vi "tb_01-x.vi"(0 "Etude":T2, 1 "Aff ?":bool, 5 "VS":T4, 7 "ent-2D":string[][](array[string]), 9 "do-2D":string[][](array[string]), 11 "tb in ?":bool[](array[boolean])) -> (4 "Etude":T2, 6 "VS":T4, 8 "ent-2D":T1[][](array[typedef]), 10 "do-2D":string[][](array[string]), 12 "X":string[](array[string]), 13 "X-ent":T1, 14 "X-lib":T1, 15 "tb in ?":bool[](array[boolean]))   [LabVIEW 2010, in "lv_04.lvlib"]
uses:
  lv_04/lv_04.lvlib
  lv_04/commandes/cX.ctl
  lv_04/commandes/cSTA_varid.ctl
  lv_04/commandes/c_TDMS_ch_variable.ctl
  lv_04/commandes/c_TDMS_ch_donnees.ctl
  lv_04/commandes/c0-var-n.ctl
  lv_04/commandes/cSTA_num_do_cr.ctl
  lv_04/commandes/c02-do-num.ctl
  lv_04/commandes/c04-stat-num.ctl
  lv_04/commandes/cSTA_txt_do_cr.ctl
  lv_04/commandes/c02-do-txt.ctl
  lv_04/commandes/c04-stat-txt.ctl
  lv_04/commandes/cSTA_dist.ctl
  lv_04/commandes/c03-dist-S.ctl
  lv_04/commandes/c0-dist-xy.ctl
  lv_04/commandes/c03-dist-T.ctl
  lv_04/commandes/c03-dist-SPC.ctl
  lv_04/commandes/c_etude.ctl
  lv_02/p_5E_ch_loi.ctl
  lv_01/type format.ctl
  lv_01/lv_01.lvlib
  lv_02/lv_02.lvlib
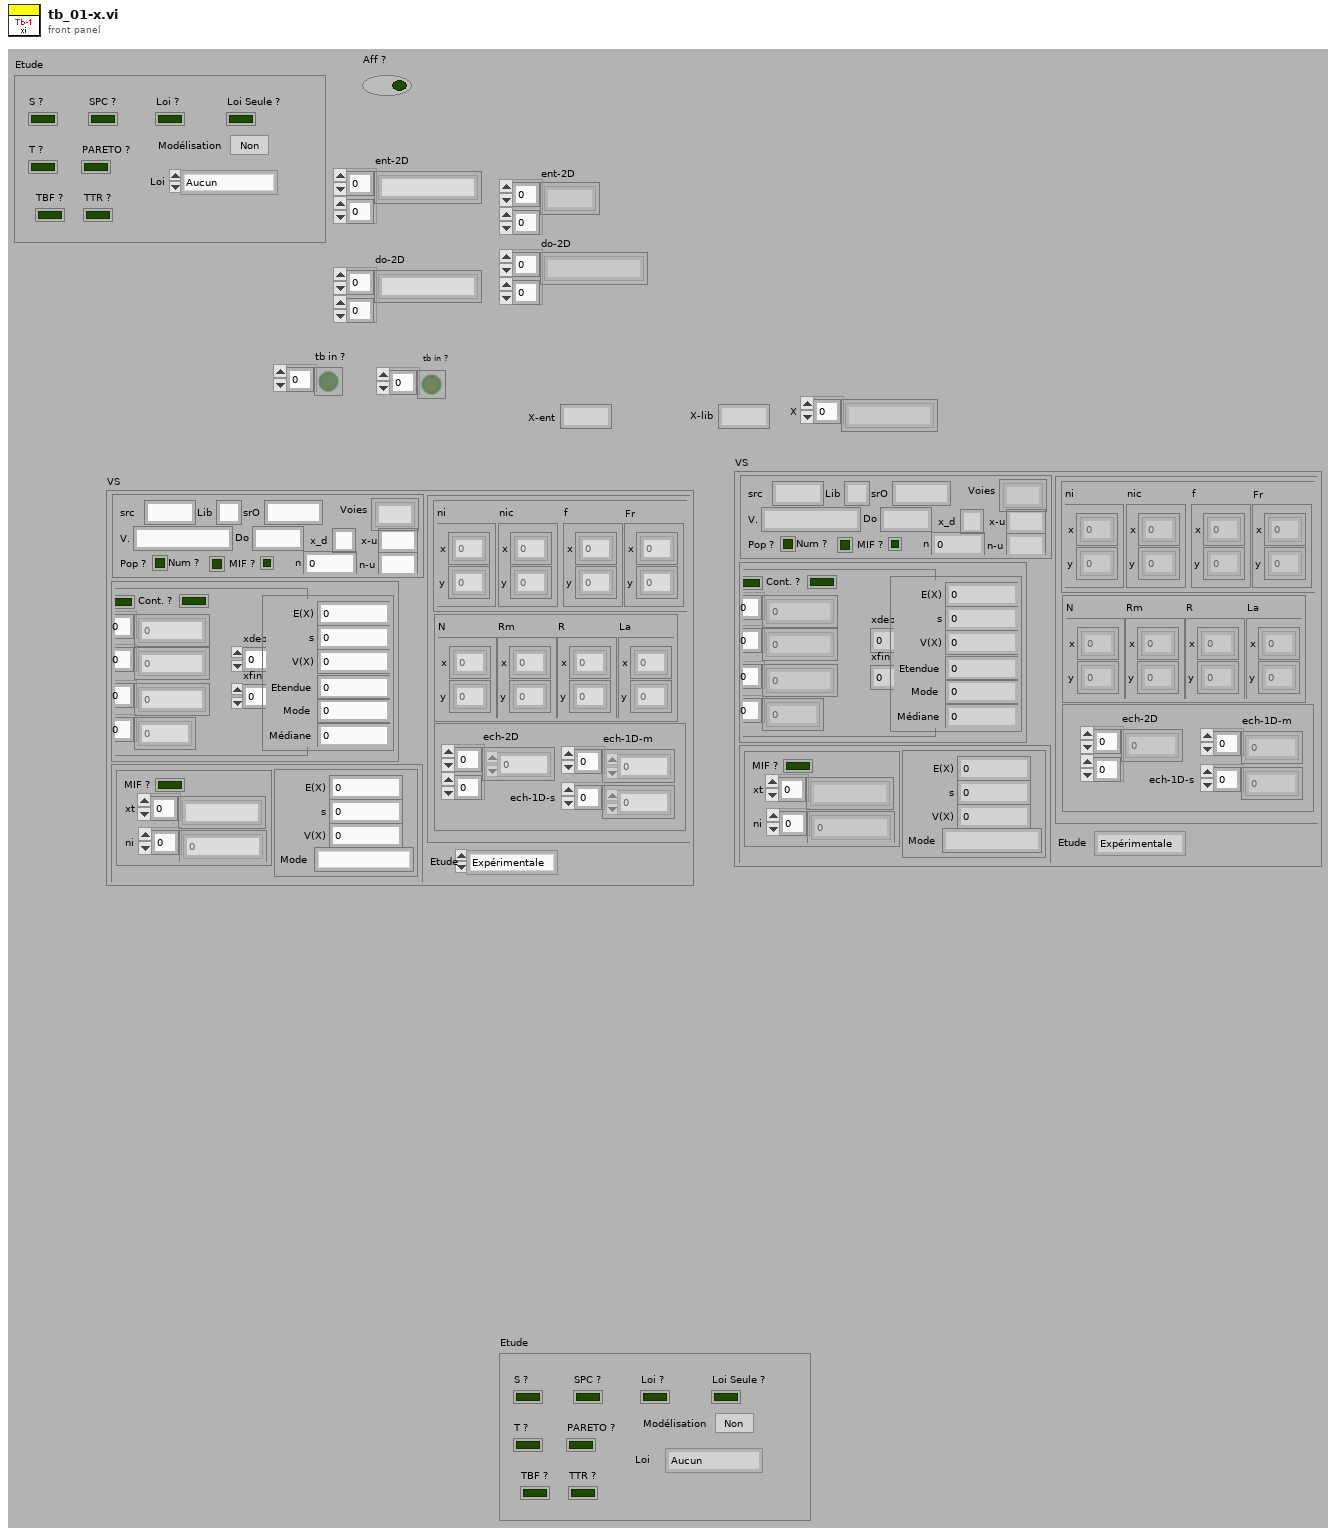
[diagram p1: front panel]
types:
  T1 = typedef "lv_04.lvlib/c_TDMS_ch_donnees.ctl" = string
  T2 = typedef "lv_04.lvlib/c_etude.ctl" = cluster{"T ?":bool, "S ?":bool, "SPC ?":bool, "PARETO ?":bool, "TBF ?":bool, "TTR ?":bool, "Loi ?":bool, "Loi Seule ?":bool, "Modélisation":bool, "Loi":T3}
  T3 = typedef "lv_02.lvlib/p_5E_ch_loi.ctl" = enum16{"Aucun", "Normale", "Aucun2", "Aucun3", "Binômial", "Poisson", "Exponentiel", "Weibull", "Rang médian"}
  T4 = typedef "lv_04.lvlib/cX.ctl" = cluster{"src":T5, "num":T8, "txt":T11, "dist":T14, "Etude":enum16{"Expérimentale", "Modèle"}}
  T5 = typedef "lv_04.lvlib/cSTA_varid.ctl" = cluster{"src":string, "Lib":string, "srO":string, "V.":T6, "Voies":string[], "Do":T1, "n":T7, "Num ?":bool, "Pop ?":bool, "x_d":string, "x-u":string, "n-u":string, "MIF ?":bool}
  T6 = typedef "lv_04.lvlib/c_TDMS_ch_variable.ctl" = string
  T7 = typedef "lv_04.lvlib/c0-var-n.ctl" = i32
  T8 = typedef "lv_04.lvlib/cSTA_num_do_cr.ctl" = cluster{"do":T9, "sta":T10}
  T9 = typedef "lv_04.lvlib/c02-do-num.ctl" = cluster{"MIF ?":bool, "Cont. ?":bool, "xi":dbl[], "xic":dbl[], "ni":u32[], "dx":dbl[], "xdeb":dbl, "xfin":dbl}
  T10 = typedef "lv_04.lvlib/c04-stat-num.ctl" = cluster{"E(X)":dbl, "s":dbl, "V(X) ":dbl, "Etendue":dbl, "Mode":dbl, "Médiane":dbl}
  T11 = typedef "lv_04.lvlib/cSTA_txt_do_cr.ctl" = cluster{"do":T12, "sta":T13}
  T12 = typedef "lv_04.lvlib/c02-do-txt.ctl" = cluster{"xt":string[], "ni":dbl[], "MIF ?":bool}
  T13 = typedef "lv_04.lvlib/c04-stat-txt.ctl" = cluster{"E(X)":dbl, "s":dbl, "V(X) ":dbl, "Mode":string}
  T14 = typedef "lv_04.lvlib/cSTA_dist.ctl" = cluster{"S":T15, "T":T17, "spc":T18}
  T15 = typedef "lv_04.lvlib/c03-dist-S.ctl" = cluster{"nic":T16, "f":T16, "Fr":T16, "ni":T16}
  T16 = typedef "lv_04.lvlib/c0-dist-xy.ctl" = cluster{"x":dbl[], "y":dbl[]}
  T17 = typedef "lv_04.lvlib/c03-dist-T.ctl" = cluster{"N":T16, "Rm":T16, "R":T16, "La":T16}
  T18 = typedef "lv_04.lvlib/c03-dist-SPC.ctl" = cluster{"ech-2D":dbl[][], "ech-1D-m":dbl[], "ech-1D-s":dbl[]}
  T19 = typedef "lv_01.lvlib/type format.ctl" = enum16{"X (dbl)", "P (Proba)", "N (entier)", "S (Scient.)"}
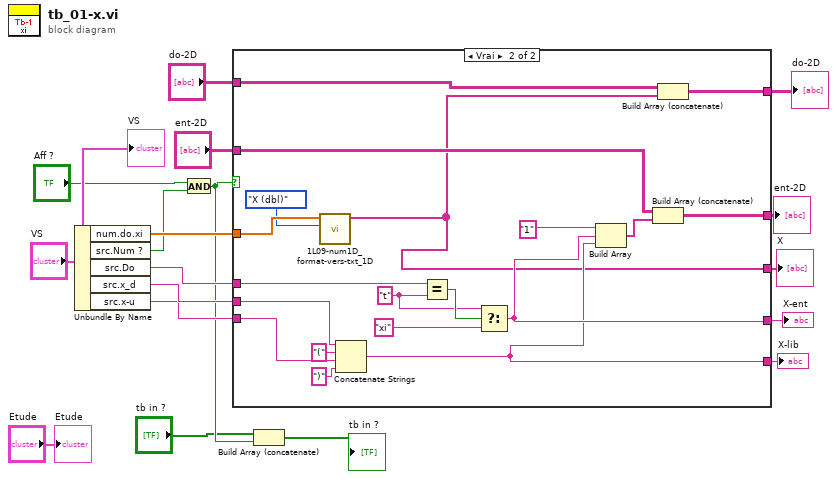
[diagram p0: block diagram]
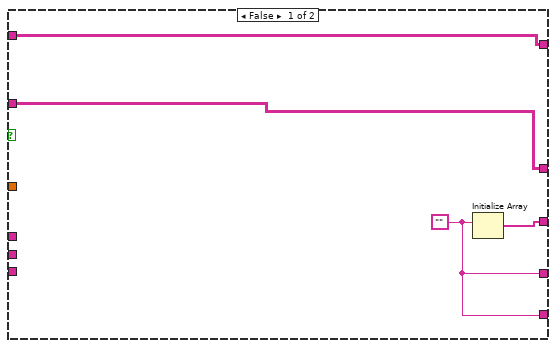
[diagram p2: hidden frame]
diagram:
  n1 = Unbundle By Name("VS") -> ("num.do.xi"=w18:dbl[], "src.Num ?"=w5:bool, "src.Do"=w7:T1, "src.x_d"=w16:string, "src.x-u"=w15:string)
  n2 = And(x="Aff ?", y=w5) -> (x .and. y?=w3:bool)
  n3 = case shown="Vrai" w3 {
    tunnel: w18 -> [_ w41]
    tunnel: w16 -> [_ w39]
    tunnel: w15 -> [_ w37]
    tunnel: [w19 w31] -> w13
    tunnel: [w19 w30] -> w12
    tunnel: "ent-2D" -> [w21 w29]
    tunnel: [w21 w27] -> w10
    tunnel: "do-2D" -> [w22 w26]
    tunnel: [w20 w23] -> w8
    tunnel: w7 -> [_ w25]
    tunnel: [w22 w24] -> w6
    frame False {
      w19 = ""
      n4 = Initialize Array(w19) -> (w20:string[])  [unwired: 1 in]
    }
    frame True {
      w34 = T1 "t" ("y")
      n5 = call "1L09-num1D_format-vers-txt_1D.vi"("type"=type_format."X (dbl)", "1D( num)"=w41) -> ("1D (ch)"=w23:string[])  [unwired: 7 in]
      n6 = Concatenate Strings(w39, "(" ("chaîne"), w37, ")" ("chaîne")) -> (w30:string)
      n7 = Equal?(x=w25, y=w34) -> (x = y?=w35:bool)
      n8 = Select(t=w34, s=w35, f=T1 "xi" ("y")) -> (s? t:f=w31:T1)
      n9 = Build Array("1", w31, w30) -> (w28:T1[])
      n10 = Build Array (concatenate)(w29, w28) -> (w27:T1[][])
      n11 = Build Array (concatenate)(w26, w23) -> (w24:string[][])
    }
  }
  "X" <- w8
  "X-ent" <- w13
  "X-lib" <- w12
  "ent-2D" <- w10
  "do-2D" <- w6
  n12 = Build Array (concatenate)("tb in ?", w3) -> (→"tb in ?":bool[])
  "VS" <- "VS"
  "Etude" <- "Etude"
